vi "ProcessClass.vi"(8 "error in (no error)":errorcluster, 10 "Blacklist Class":T1, 11 "VI Refnum":refnum<vi>) -> (0 "error out":errorcluster, 1 "Output/Failure":string, 2 "Reject?":bool, 3 "dup VI Refnum":refnum<vi>)   [LabVIEW 2014, in "BuildSecurity.lvlib"]
doc: "Checks for a specific class of blacklisted items. If an item is found, <b>Reject?</b> will return <b>TRUE</b>."
uses:
  BuildSecurity.lvlib
  BlacklistClassInfo.ctl
  Blacklist/Blacklist.lvclass
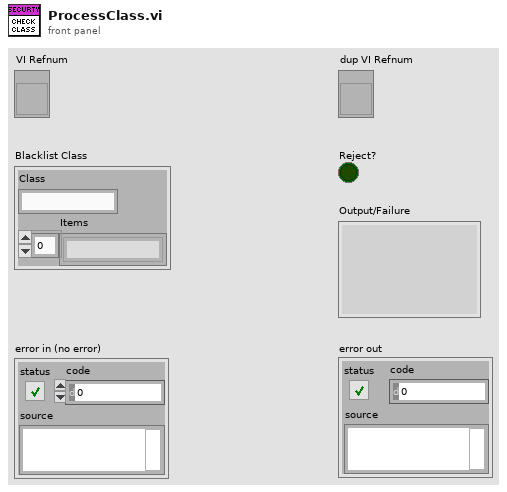
[diagram p1: front panel]
types:
  T1 = typedef "BuildSecurity.lvlib/BlacklistClassInfo.ctl" = cluster{"Class":string, "Items":string[]}
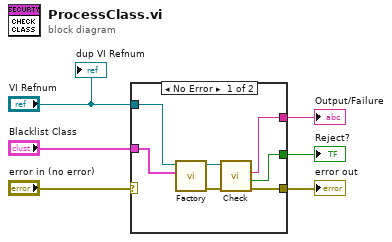
[diagram p0: block diagram]
diagram:
  n1 = case shown="No Error" "error in (no error)" {
    selector: "error in (no error)" -> [_ w14]
    tunnel: "Blacklist Class" -> [w13 _]
    tunnel: [w9 w14] -> w4
    tunnel: "VI Refnum" -> [w10 _]
    tunnel: [w8 _] -> w2
    tunnel: [w7 _] -> w1
    frame No Error {
      n2 = call "Factory.vi"("Blacklist Class"=w13, "VI Refnum"=w10) -> ("error out"=w12:errorcluster, "Blacklist out"=w11:refnum<class "Blacklist.lvclass">)  [unwired: 8 in]
      n3 = call "Check.vi"("error in (no error)"=w12, "Blacklist in"=w11) -> ("error out"=w9:errorcluster, "Reject?"=w7:bool, "Output"=w8:string)  [unwired: 6 in, 1 out]
    }
    frame Error {
    }
  }
  "error out" <- w4
  "Reject?" <- w1
  "Output/Failure" <- w2
  "dup VI Refnum" <- "VI Refnum"
